vi "Main RT.vi"   [LabVIEW 2025]
uses:
  <vilib>/FPGAPlugInAG/myRIO-1900/niLvFpga_Open_myRIO-1900.vi
  <vilib>/rvi/interface/common/dynamic/niFpgaDynamicAddResources.vi
  <vilib>/Utility/error.llb/Error Cluster From Error Code.vi
  <vilib>/rvi/errors/niLvFpgaAdjustHostInterfaceError.vi
  <vilib>/FPGAPlugInAG/Dynamic/niLvFpga_Close_Dynamic.vi
  <vilib>/rvi/interface/nirviOpenFPGA/nirviOpenFPGA.xnode
  FPGA Bitfiles/myriofpga_FPGATarget_MainFPGA_jtfUHSB2PLk.lvbitx
  <vilib>/rvi/interface/nirviReadWriteControl/nirviReadWriteControl.xnode
  <vilib>/rvi/interface/nirviCloseFPGA/nirviCloseFPGA.xnode
  NiFpgaLv.dll
  <vilib>/rvi/interface/Simulation/niFpgaSimulationCallBeginRW.vi
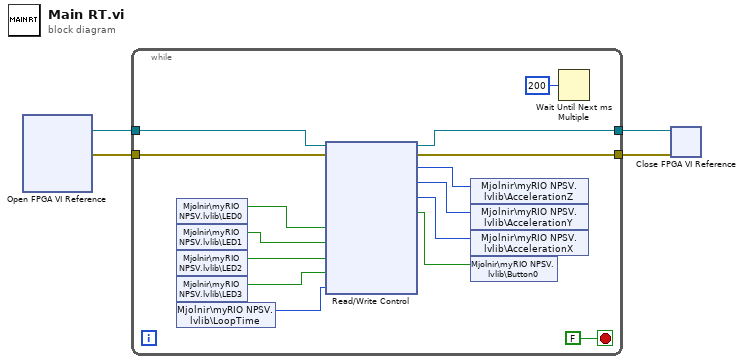
[diagram p0: block diagram]
diagram:
  n1 = xnode "Open FPGA VI Reference"() -> ("FPGA VI Reference Out"=w2:refnum<k20>, "error out"=w4:errorcluster)  [unwired: 2 in]
  n2 = while {
    tunnel: w4 -> [w18]
    tunnel: [w17] -> w3
    tunnel: w2 -> [w19]
    tunnel: [w16] -> w1
    stop <- FALSE stop-if-true
    n3 = shared-variable "Mjolnir\\myRIO NPSV.lvlib\\LED0"() -> (w11:bool)  [unwired: 1 in, 1 out]
    n4 = shared-variable "Mjolnir\\myRIO NPSV.lvlib\\LED1"() -> (w12:bool)  [unwired: 1 in, 1 out]
    n5 = shared-variable "Mjolnir\\myRIO NPSV.lvlib\\LED2"() -> (w13:bool)  [unwired: 1 in, 1 out]
    n6 = shared-variable "Mjolnir\\myRIO NPSV.lvlib\\LED3"() -> (w14:bool)  [unwired: 1 in, 1 out]
    n7 = shared-variable "Mjolnir\\myRIO NPSV.lvlib\\LoopTime"() -> (w15:u32)  [unwired: 1 in, 1 out]
    n8 = xnode "Read/Write Control"("FPGA VI Reference In"=w19, "error in"=w18, "LED0"=w11, "LED1"=w12, "LED2"=w13, "LED3"=w14, "Count(mSec)"=w15) -> ("FPGA VI Reference Out"=w16:refnum<k20>, "error out"=w17:errorcluster, "AccelerationZ"=w10:i16, "AccelerationY"=w9:i16, "AccelerationX"=w8:i16, "Button0"=w7:bool)
    n9 = shared-variable "Mjolnir\\myRIO NPSV.lvlib\\AccelerationZ"(w10) -> ()  [unwired: 1 in, 1 out]
    n10 = shared-variable "Mjolnir\\myRIO NPSV.lvlib\\AccelerationY"(w9) -> ()  [unwired: 1 in, 1 out]
    n11 = shared-variable "Mjolnir\\myRIO NPSV.lvlib\\AccelerationX"(w8) -> ()  [unwired: 1 in, 1 out]
    n12 = shared-variable "Mjolnir\\myRIO NPSV.lvlib\\Button0"(w7) -> ()  [unwired: 1 in, 1 out]
    n13 = Wait Until Next ms Multiple(millisecond multiple=u32 200) -> ()  [unwired: 1 out]
  }
  n14 = xnode "Close FPGA VI Reference"("FPGA VI Reference In"=w1, "error in"=w3) -> ()  [unwired: 1 out]
